vi "Convert Double EOL.vi"(9 "convert to":string, 10 "string in":string) -> (2 "string out":string)   [LabVIEW 2019, in "MD Generator.lvlib"]
uses:
  MD Generator.lvlib
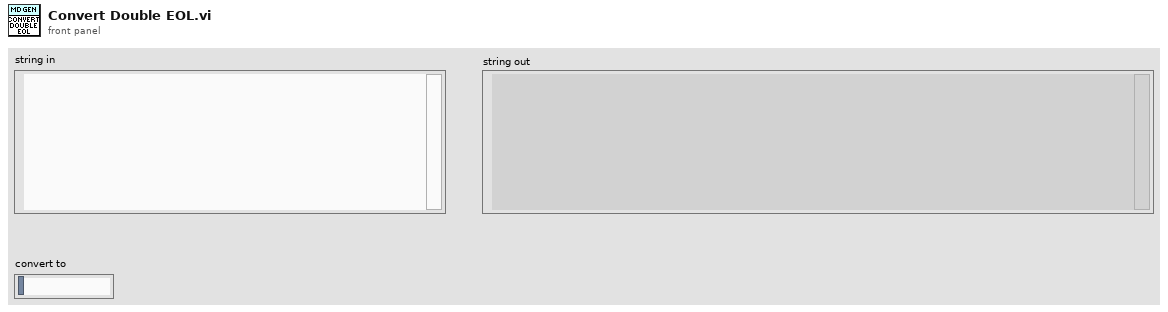
[diagram p1: front panel]
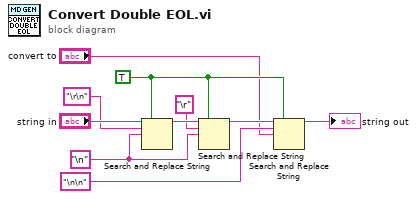
[diagram p0: block diagram]
diagram:
  w6 = TRUE ("replace all? (F)")
  w4 = "\n" ("search string")
  n1 = Search and Replace String(replace all?=w6, input string="string in", search string="\r\n", replace string=w4) -> (result string=w9:string)  [unwired: 4 in, 3 out]
  n2 = Search and Replace String(replace all?=w6, input string=w9, search string="\r", replace string=w4) -> (result string=w7:string)  [unwired: 4 in, 3 out]
  n3 = Search and Replace String(replace all?=w6, input string=w7, search string="\n\n", replace string="convert to") -> (result string=→"string out":string)  [unwired: 4 in, 3 out]
